vi "rx_close.vi"(8 "error in":errorcluster, 10 "Queues":T1, 11 "HW parameters":T2={"Device IP Address"="192.168.11.6", "Active Antenna"="RX1", "Carrier Frequency (Hz)"=915000000.0, "Gain (dB)"=10.0, "Trigger Level"=0.01, "Bandwidth (Hz)"=40000000.0, "Reference Position (%)"=10.0, "Capture Time (s)"=0.0004, "Simulate"=FALSE} {"Capture Time (s)" format="%.2p"; "Bandwidth (Hz)" format="%.2p"; "Trigger Level" format="%#.3p"; "Gain (dB)" format="%.2f"; "Carrier Frequency (Hz)" format="%.2p"}) -> (0 "error out":errorcluster)   [LabVIEW 2012, in "gds_hw_config.lvlib"]
uses:
  EE 497/LABS/SDR/control_type_defs.llb/rx_hw params.ctl
  EE 497/LABS/SDR/control_type_defs.llb/Queues.ctl
  gds_hw_config.lvlib
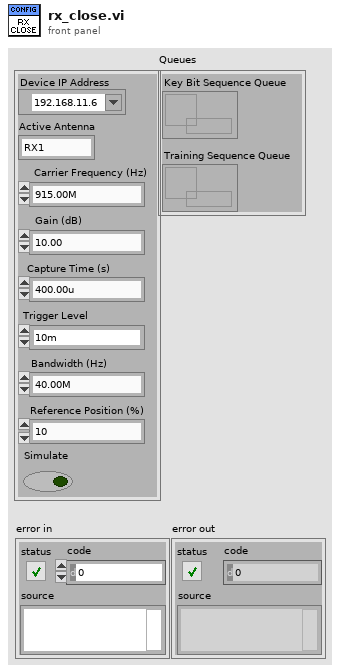
[diagram p1: front panel]
types:
  T1 = typedef "Queues.ctl" = cluster{"Key Bit Sequence Queue":refnum<queue>, "Training Sequence Queue":refnum<queue>}
  T2 = typedef "rx_hw params.ctl" = cluster{"Device IP Address":refnum<k15>, "Active Antenna":string, "Carrier Frequency (Hz)":dbl, "Gain (dB)":dbl, "Trigger Level":dbl, "Bandwidth (Hz)":dbl, "Reference Position (%)":dbl, "Capture Time (s)":dbl, "Simulate":bool}
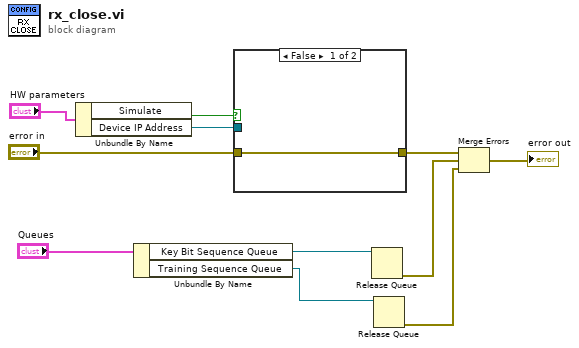
[diagram p0: block diagram]
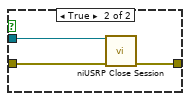
[diagram p2: hidden frame]
diagram:
  n1 = Unbundle By Name("HW parameters") -> ("Simulate"=w10:bool, "Device IP Address"=w9:refnum<k15>)
  n2 = Unbundle By Name("Queues") -> ("Key Bit Sequence Queue"=w6:refnum<queue>, "Training Sequence Queue"=w5:refnum<queue>)
  n3 = case shown="False" w10 {
    tunnel: w9 -> [_ w15]
    tunnel: "error in" -> [w12 w14]
    tunnel: [w12 w13] -> w4
    frame False {
    }
    frame True {
      n4 = call <instrlib>:"niUSRP Close Session.vi"("session handle"=w15, "error in (no error)"=w14) -> ("error out"=w13:errorcluster)  [unwired: 13 in]
    }
  }
  n5 = Release Queue(queue=w6) -> (error out=w3:errorcluster)  [unwired: 2 in, 2 out]
  n6 = Release Queue(queue=w5) -> (error out=w2:errorcluster)  [unwired: 2 in, 2 out]
  n7 = Merge Errors(w4, w3, w2) -> (→"error out":errorcluster)
